vi "LVClass_Camera get Parameter Values SetAndGet.vi"(0 "Camera in":refnum<class "Camera.lvclass">, 11 "error in (no error)":errorcluster) -> (4 "Camera out":refnum<class "Camera.lvclass">, 6 "ListOfSettableAndGettableValue":T1[](array[typedef]), 10 "BG Image OUT":refnum<class "Image.lvclass">, 15 "error out":errorcluster)   [LabVIEW 2020, in "Camera.lvclass"]
doc: "Get camera parameters which are gettable and settable parameter \n\n<B>CameraIn</B> : Camera object.\n<B>CameraOut</B> : Camera object.\n<B>BG Image OUIT</B> : Defined background image object if it is allready defined throught camera object method \"LVClass_Camera set background.vi\".\nThis image object is a reference : DO NOT DELETE THIS OBJECT BY YOURSELF\n<B>ListOfSettableAndGettableValue</B> : Array of the parameter with readen value from camera object."
uses:
  Camera.lvclass
  CameraParametersSetup.ctl
  CameraParameters_Type.ctl
  Image.lvclass
  Camera.lvclass/Camera.ctl
  LVClass_Camera Read acquisition state.vi
  LVClass_Camera Read all camera parameters.vi
  LVClass_Image read Image Compat ptr.vi
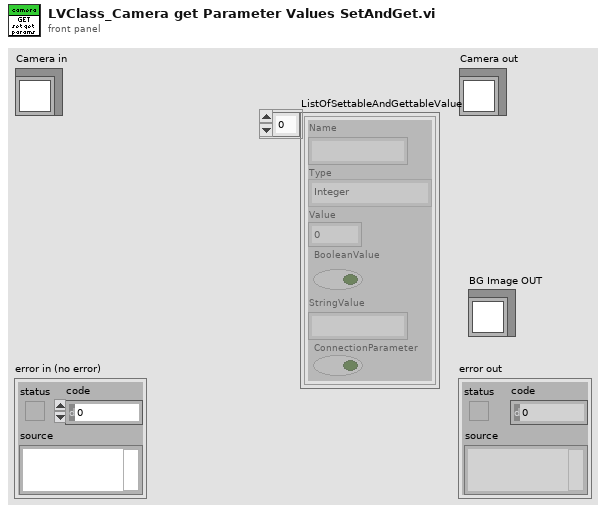
[diagram p1: front panel]
types:
  T1 = typedef "CameraParametersSetup.ctl" = cluster{"Name":string, "Type":T2, "Value":dbl, "BooleanValue":bool, "StringValue":string, "ConnectionParameter":bool}
  T2 = typedef "CameraParameters_Type.ctl" = enum16{"Integer", "Real", "String", "Boolean"}
  T3 = typedef "CameraAcquisitionState.ctl" = enum16{"Stop", "Live"}
  T4 = typedef "ParameterID.ctl" = cluster{"Name":string, "ConnectionParameter?":bool, "Type":T2, "Authorization":T5, "OnFlyAuthorization":T6, "StringValue":string, "Value":dbl, "Min":dbl, "Max":dbl, "BooleanValue":bool, "StringParameterList":string[]}
  T5 = typedef "CameraParameters_Authorization.ctl" = enum16{"Disable", "Gettable", "Settable - Gettable"}
  T6 = typedef "CameraParameters_OnFlyAuthorization.ctl" = enum16{"None", "Gettable", "Settable", "Settable - Gettable"}
  T7 = typedef "ClassID.ctl" = i64
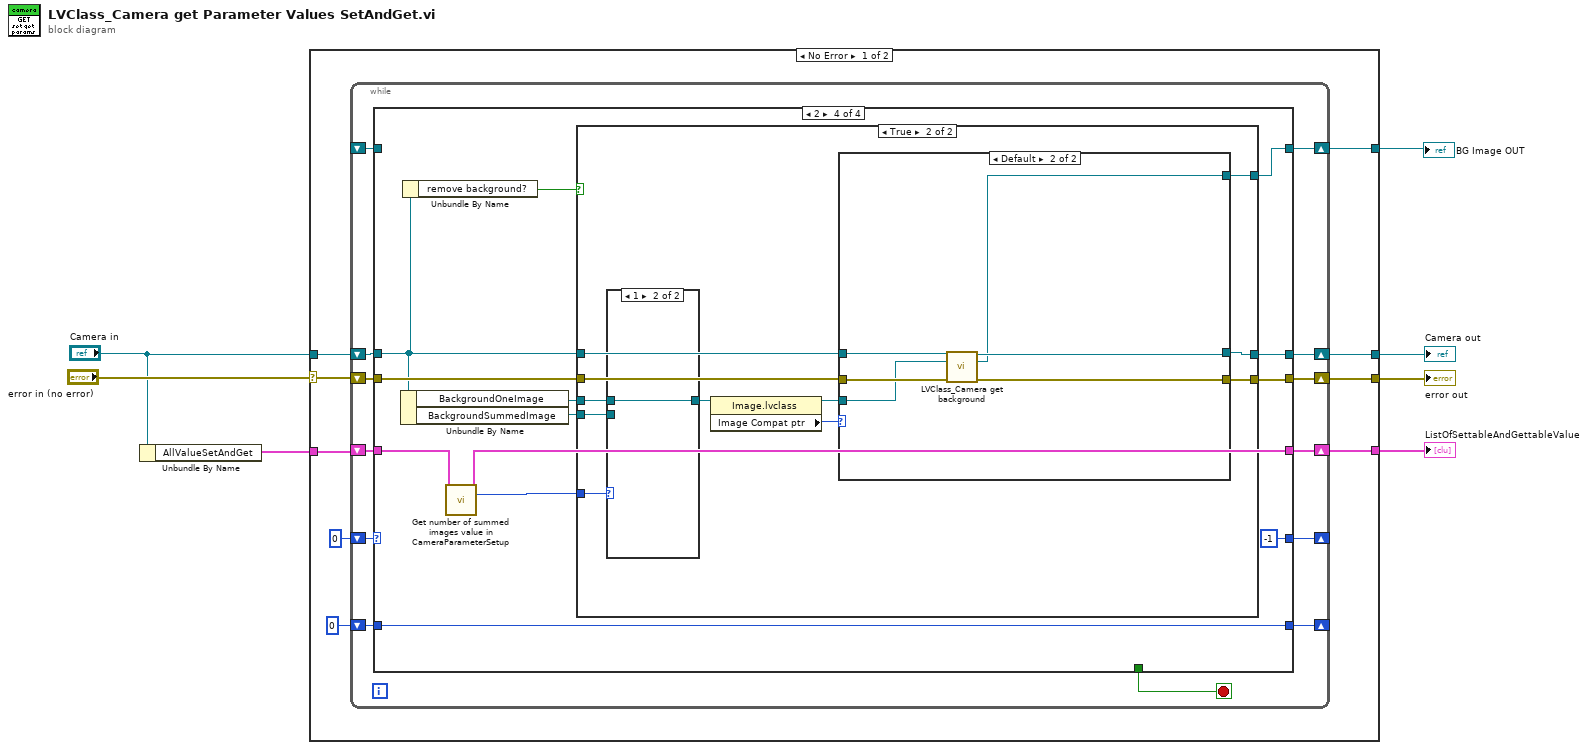
[diagram p0: block diagram]
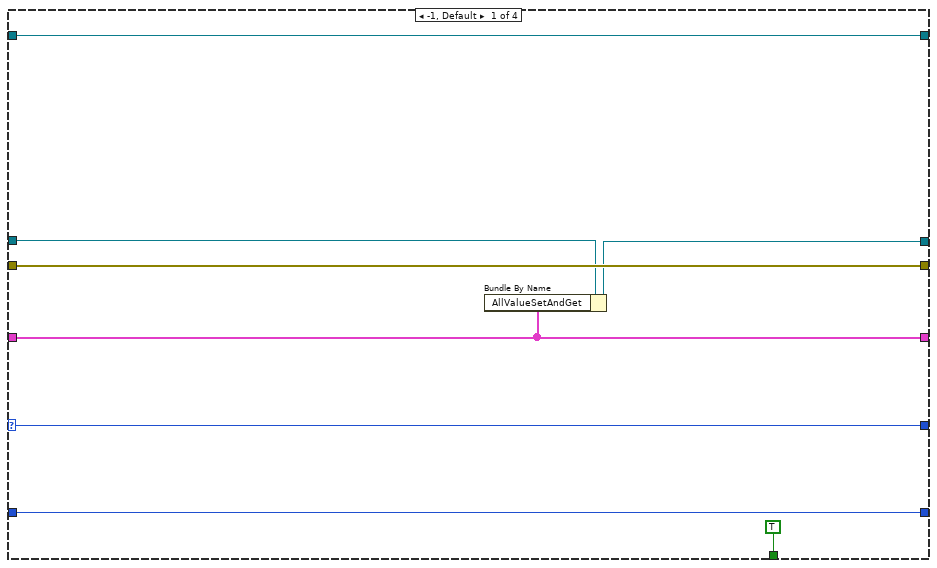
[diagram p2: hidden frame]
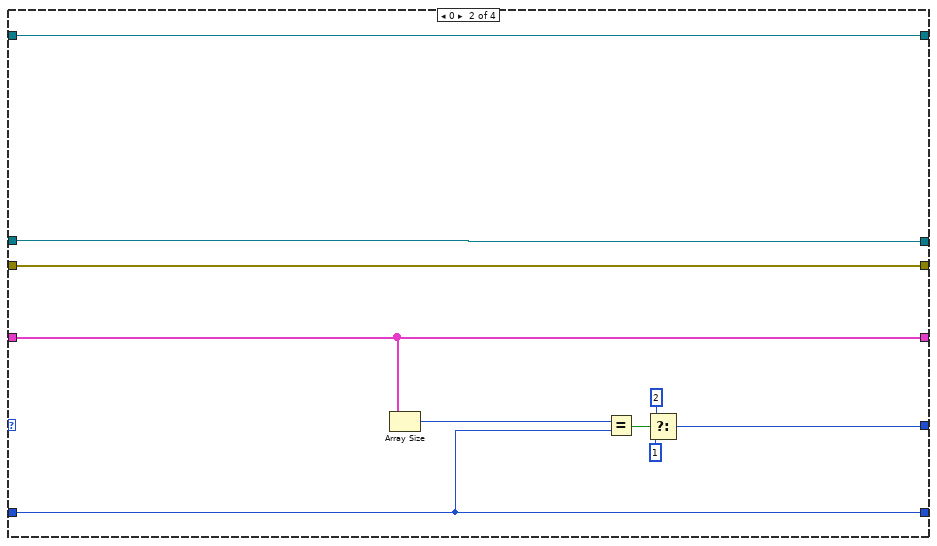
[diagram p3: hidden frame]
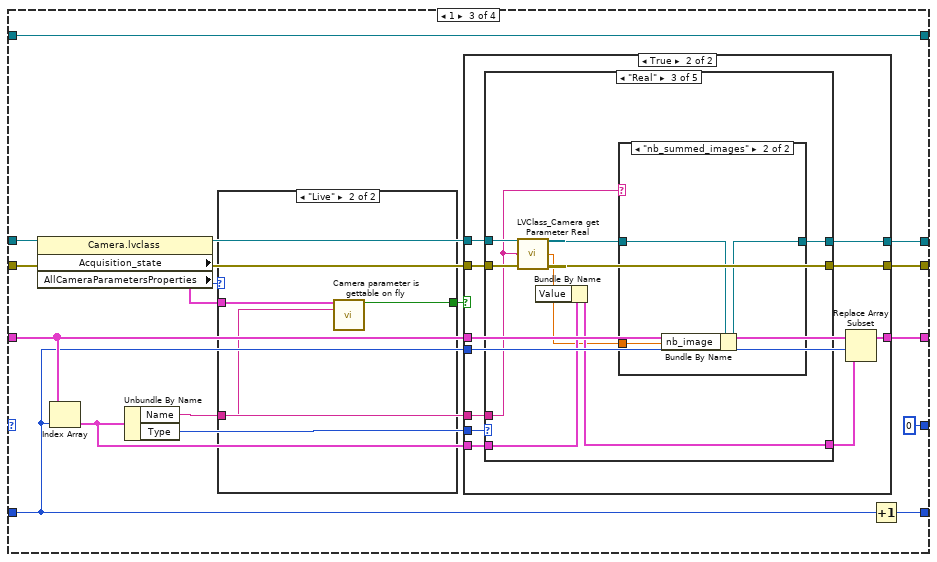
[diagram p4: hidden frame]
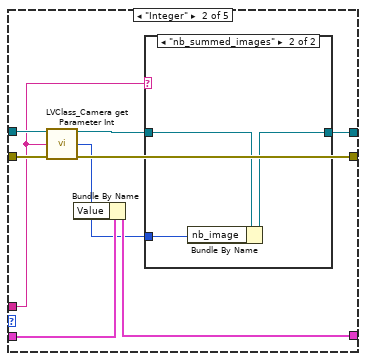
[diagram p7: hidden frame]
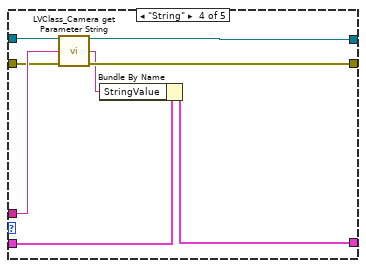
[diagram p10: hidden frame]
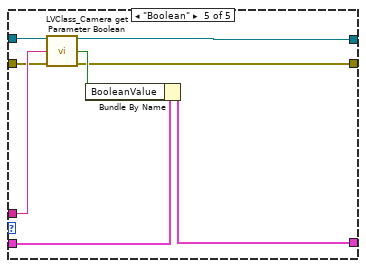
[diagram p11: hidden frame]
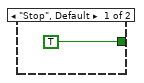
[diagram p12: hidden frame]
diagram:
  n1 = Unbundle By Name("Camera in") -> ("AllValueSetAndGet"=w1:T1[])
  n2 = case shown="No Error" "error in (no error)" {
    selector: "error in (no error)" -> [w12 w168]
    tunnel: [w13 w168] -> w6
    tunnel: [w14 w167] -> w5
    tunnel: "Camera in" -> [w16 w167]
    tunnel: [w11 _] -> w4
    tunnel: [w10 _] -> w3
    tunnel: w1 -> [w8 _]
    frame No Error {
      n3 = while {
        shift-right: [w28] -> _
        shift-left: 0 -> [w27]
        shift-right: [w25] -> w13
        shift-left: w12 -> [w24]
        shift-right: [w26] -> w14
        shift-left: w16 -> [w29]
        shift-right: [w21] -> w11
        shift-left: _ -> [w22]
        shift-right: [w20] -> w10
        shift-left: w8 -> [w19]
        shift-right: [w17] -> _
        shift-left: 0 -> [w18]
        stop <- w23 stop-if-true
        n4 = case shown="2" w27 {
          selector: w27 -> [w33 _ _ _]
          tunnel: w29 -> [w32 w47 w55 w136]
          tunnel: w24 -> [w36 w46 w53 w141]
          tunnel: [w33 w39 0 -1] -> w28
          tunnel: [w31 w47 w64 w140] -> w26
          tunnel: [w36 w46 w63 w139] -> w25
          tunnel: [TRUE _ _ _] -> w23
          tunnel: w22 -> [w35 w45 w62 _]
          tunnel: [w35 w45 w62 w138] -> w21
          tunnel: [w30 w44 w57 w130] -> w20
          tunnel: w19 -> [w30 w44 w59 w131]
          tunnel: w18 -> [w34 w42 w58 w132]
          tunnel: [w34 w42 w61 w132] -> w17
          frame -1, Default {
            n5 = Bundle By Name(cluster=w32, "AllValueSetAndGet"=w30) -> (w31:refnum<class "Camera.lvclass">)
          }
          frame 0 {
            n6 = Array Size(array=w44) -> (size(s)=w43:i32)
            n7 = Equal?(x=w43, y=w42) -> (x = y?=w41:bool)
            n8 = Select(t=2, s=w41, f=1) -> (s? t:f=w39:i32)
          }
          frame 1 {
            n9 = property class="Camera.lvclass"(reference=w55, error in=w53) -> (reference out=w54:refnum<class "Camera.lvclass">, error out=w52:errorcluster, "Acquisition_state"=w51:T3, "AllCameraParametersProperties"=w50:T4[])
            n10 = Index Array(array=w59, index=w58) -> (element=w60:T1)
            n11 = Unbundle By Name(w60) -> ("Name"=w48:string, "Type"=w56:T2)
            n12 = case shown="\"Live\"" w51 {
              tunnel: w50 -> [_ w127]
              tunnel: [TRUE w128] -> w49
              tunnel: w48 -> [_ w126]
              frame "Stop", Default {
              }
              frame "Live" {
                n13 = call "Camera parameter is gettable on fly.vi"("AllCameraParameters"=w127, "Name"=w126) -> ("Gettable?"=w128:bool)  [unwired: 13 in]
              }
            }
            n14 = case shown="True" w49 {
              tunnel: [w68 w79] -> w64
              tunnel: [w67 w78] -> w63
              tunnel: w60 -> [_ w77]
              tunnel: w59 -> [w66 w76]
              tunnel: w58 -> [_ w75]
              tunnel: [w66 w74] -> w57
              tunnel: w56 -> [_ w73]
              tunnel: w48 -> [_ w72]
              tunnel: w54 -> [w68 w71]
              tunnel: w52 -> [w67 w70]
              frame False {
              }
              frame True {
                n15 = case shown="\"Real\"" w73 {
                  tunnel: w77 -> [w80 w91 w100 w109 w118]
                  tunnel: [w80 w90 w101 w116 w117] -> w69
                  tunnel: w72 -> [_ w83 w99 w113 w123]
                  tunnel: w71 -> [w82 w89 w104 w115 w124]
                  tunnel: [w82 w85 w96 w114 w121] -> w79
                  tunnel: [w81 w88 w102 w111 w119] -> w78
                  tunnel: w70 -> [w81 w87 w103 w112 w122]
                  frame Default {
                  }
                  frame "Integer" {
                    n16 = call "LVClass_Camera get Parameter Int.vi"("Camera in"=w89, "parameter_name"=w83, "error in (no error)"=w87) -> ("Camera out"=w86:refnum<class "Camera.lvclass">, "value"=w84:i32, "error out"=w88:errorcluster)  [unwired: 10 in]
                    n17 = Bundle By Name(cluster=w91, "Value"=w84) -> (w90:T1)
                    n18 = case shown="\"nb_summed_images\"" w83 {
                      tunnel: [w92 w94] -> w85
                      tunnel: w86 -> [w92 w95]
                      tunnel: w84 -> [_ w93]
                      frame Default {
                      }
                      frame "nb_summed_images" {
                        n19 = Bundle By Name(cluster=w95, "nb_image"=w93) -> (w94:refnum<class "Camera.lvclass">)
                      }
                    }
                  }
                  frame "Real" {
                    n20 = call "LVClass_Camera get Parameter Real.vi"("Camera in"=w104, "parameter_name"=w99, "error in (no error)"=w103) -> ("Camera out"=w97:refnum<class "Camera.lvclass">, "value"=w98:dbl, "error out"=w102:errorcluster)  [unwired: 10 in]
                    n21 = Bundle By Name(cluster=w100, "Value"=w98) -> (w101:T1)
                    n22 = case shown="\"nb_summed_images\"" w99 {
                      tunnel: [w105 w107] -> w96
                      tunnel: w97 -> [w105 w108]
                      tunnel: w98 -> [_ w106]
                      frame Default {
                      }
                      frame "nb_summed_images" {
                        n23 = Bundle By Name(cluster=w108, "nb_image"=w106) -> (w107:refnum<class "Camera.lvclass">)
                      }
                    }
                  }
                  frame "String" {
                    n24 = call "LVClass_Camera get Parameter String.vi"("Camera in"=w115, "parameter_name"=w113, "error in (no error)"=w112) -> ("Camera out"=w114:refnum<class "Camera.lvclass">, "value"=w110:string, "error out"=w111:errorcluster)  [unwired: 10 in]
                    n25 = Bundle By Name(cluster=w109, "StringValue"=w110) -> (w116:T1)
                  }
                  frame "Boolean" {
                    n26 = call "LVClass_Camera get Parameter Boolean.vi"("Camera in"=w124, "parameter_name"=w123, "error in (no error)"=w122) -> ("Camera out"=w121:refnum<class "Camera.lvclass">, "value"=w120:bool, "error out"=w119:errorcluster)  [unwired: 10 in]
                    n27 = Bundle By Name(cluster=w118, "BooleanValue"=w120) -> (w117:T1)
                  }
                }
                n28 = Replace Array Subset(array=w76, new element=w69, index=w75) -> (w74:T1[])
              }
            }
            n29 = Increment(x=w58) -> (x+1=w61:i32)
          }
          frame 2 {
            n30 = Unbundle By Name(w136) -> ("BackgroundOneImage"=w137:refnum<class "Image.lvclass">, "BackgroundSummedImage"=w133:refnum<class "Image.lvclass">)
            n31 = Unbundle By Name(w136) -> ("remove background?"=w134:bool)
            n32 = call "Get number of summed images value in CameraParameterSetup.vi"("CameraParametersSetup"=w131) -> ("CameraParametersSetup (dup)"=w130:T1[], "nb_summed_images"=w129:i32)  [unwired: 13 in]
            n33 = case shown="True" w134 {
              tunnel: w141 -> [w142 w154]
              tunnel: [w143 w153] -> w140
              tunnel: [w142 w152] -> w139
              tunnel: [w144 w151] -> w138
              tunnel: w137 -> [w144 w147]
              tunnel: w136 -> [w143 w150]
              tunnel: w129 -> [_ w148]
              tunnel: w133 -> [_ w145]
              frame False {
              }
              frame True {
                n34 = case shown="1" w148 {
                  tunnel: w147 -> [_ w157]
                  tunnel: [w156 w157] -> w146
                  tunnel: w145 -> [w156 _]
                  frame 0, Default {
                  }
                  frame 1 {
                  }
                }
                n35 = property class="Image.lvclass"(reference=w146) -> (reference out=w149:refnum<class "Image.lvclass">, "Image Compat ptr"=w155:T7)  [unwired: 1 in, 1 out]
                n36 = case shown="Default" w155 {
                  tunnel: w150 -> [w159 w166]
                  tunnel: w154 -> [w160 w165]
                  tunnel: [w159 w164] -> w153
                  tunnel: [w160 w163] -> w152
                  tunnel: [w158 w162] -> w151
                  tunnel: w149 -> [w158 w161]
                  frame 0 {
                  }
                  frame Default {
                    n37 = call "LVClass_Camera get background.vi"("Camera in"=w166, "BG Image IN"=w161, "error in (no error)"=w165) -> ("Camera out"=w164:refnum<class "Camera.lvclass">, "BG Image OUT"=w162:refnum<class "Image.lvclass">, "error out"=w163:errorcluster)  [unwired: 10 in]
                  }
                }
              }
            }
          }
        }
      }
    }
    frame Error {
    }
  }
  "error out" <- w6
  "Camera out" <- w5
  "ListOfSettableAndGettableValue" <- w3
  "BG Image OUT" <- w4
